vi "Knob Turn.vi"(0 "GEA2 Reference In":refnum<k24>, 7 "Knob Postiton":T1=enum."Position 1", 11 "Error In":errorcluster) -> (4 "GEA2 Reference Out":refnum<k24>, 15 "Error Out":errorcluster)   [LabVIEW 2016, in "TLMB.lvlib"]
uses:
  Projects/TLMB.lvlib
  type defs/Encoder Position.ctl
  Q:/Common/DLLs/GEA3/GeaCommunication.dll
  Common/DLLs/GEA3/GeaCommunication.dll
  Common/LabVIEW GEA2 Toolkit/LabVIEW_GEA2_Toolkit.lvlibp/type defs/Source_Destination.ctl
  Common/LabVIEW GEA2 Toolkit/LabVIEW_GEA2_Toolkit.lvlibp/type defs/ERD Write Data In.ctl
  Common/LabVIEW GEA2 Toolkit/LabVIEW_GEA2_Toolkit.lvlibp/type defs/Data Type.ctl
  Common/LabVIEW GEA2 Toolkit/LabVIEW_GEA2_Toolkit.lvlibp
panel:
  in  "Standalone?":bool
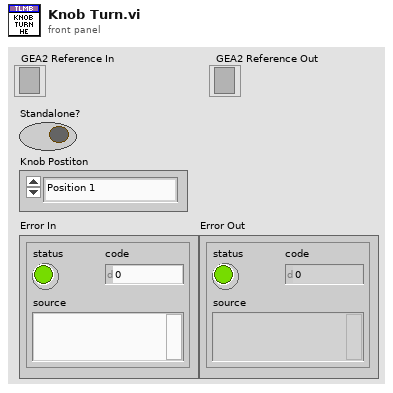
[diagram p1: front panel]
types:
  T1 = typedef "TLMB.lvlib/Encoder Position.ctl" = enum16{"Position 0", "Position 1", "Position 2", "Position 3", "Position 4", "Position 5", "Position 6", "Position 7", "Position 8", "Position 9", "Position 10", "Position 11", "Position 12", "Position 13", "Clear / Reset"}
  T2 = typedef "LabVIEW_GEA2_Toolkit.lvlibp/ERD Write Data In.ctl" = cluster{"ERD Number":u16, "Data Type":T3, "Data":string}
  T3 = typedef "LabVIEW_GEA2_Toolkit.lvlibp/Data Type.ctl" = enum16{"string", "boolean", "uint8_t", "uint16_t", "uint32_t", "uint64_t", "int8_t", "int16_t", "int32_t", "int64_t"}
  T4 = typedef "LabVIEW_GEA2_Toolkit.lvlibp/Source_Destination.ctl" = cluster{"Source":u8, "Destination":u8}
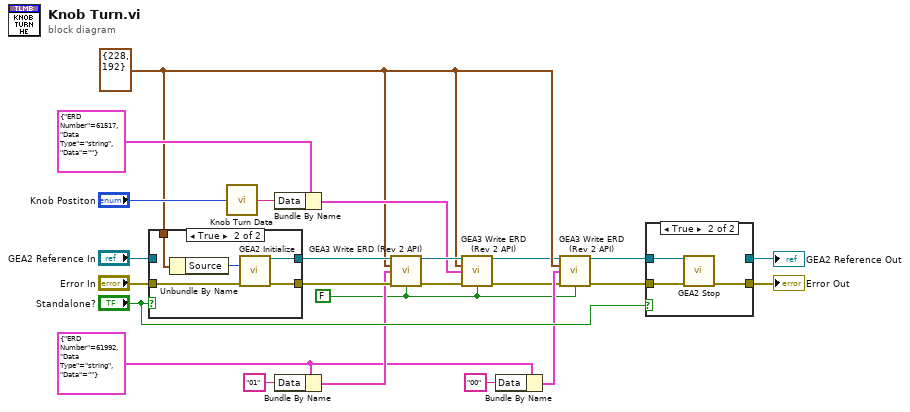
[diagram p0: block diagram]
diagram:
  w9 = T2 {"ERD Number"=61992, "Data Type"=enum."string", "Data"=""} ("ERD Write Data In")
  w4 = FALSE ("Verify ERD Response?")
  w3 = T4 {"Source"=228, "Destination"=192} ("GEA Inputs")
  n1 = case shown="True" "Standalone?" {
    tunnel: "Error In" -> [w25 w31]
    tunnel: [w25 w30] -> w17
    tunnel: "GEA2 Reference In" -> [w26 _]
    tunnel: [w26 w29] -> w18
    tunnel: w3 -> [_ w27]
    frame False {
    }
    frame True {
      n2 = Unbundle By Name(w27) -> ("Source"=w28:u8)
      n3 = call "GEA2 Initialize.vi"("Source Address"=w28, "error in"=w31) -> ("GEA2 Reference Out"=w29:refnum<k24>, "error out"=w30:errorcluster)  [unwired: 11 in, 1 out]
    }
  }
  n4 = call "Knob Turn Data.vi"("Switch"="Knob Postiton") -> ("Switch Message"=w6:string)  [unwired: 14 in]
  n5 = Bundle By Name(cluster=T2 {"ERD Number"=61517, "Data Type"=enum."string", "Data"=""} ("ERD Write Data In"), "Data"=w6) -> (w14:T2)
  n6 = Bundle By Name(cluster=w9, "Data"="01") -> (w12:T2)
  n7 = call "GEA3 Write ERD (Rev 2 API).vi"("GEA2 Reference In"=w18, "GEA Inputs"=w3, "ERD Write Data In"=w12, "Error In"=w17, "Verify ERD Response?"=w4) -> ("GEA2 Reference Out"=w16:refnum<k24>, "Error Out"=w15:errorcluster)  [unwired: 8 in, 1 out]
  n8 = call "GEA3 Write ERD (Rev 2 API).vi"("GEA2 Reference In"=w16, "GEA Inputs"=w3, "ERD Write Data In"=w14, "Error In"=w15, "Verify ERD Response?"=w4) -> ("GEA2 Reference Out"=w2:refnum<k24>, "Error Out"=w1:errorcluster)  [unwired: 8 in, 1 out]
  n9 = Bundle By Name(cluster=w9, "Data"="00") -> (w7:T2)
  n10 = call "GEA3 Write ERD (Rev 2 API).vi"("GEA2 Reference In"=w2, "GEA Inputs"=w3, "ERD Write Data In"=w7, "Error In"=w1, "Verify ERD Response?"=w4) -> ("GEA2 Reference Out"=w11:refnum<k24>, "Error Out"=w10:errorcluster)  [unwired: 8 in, 1 out]
  n11 = case shown="True" "Standalone?" {
    tunnel: [w32 w36] -> w21
    tunnel: w11 -> [w33 w35]
    tunnel: [w33 _] -> w20
    tunnel: w10 -> [w32 w34]
    frame False {
    }
    frame True {
      n12 = call "GEA2 Stop.vi"("GEA2 Reference In"=w35, "Error In"=w34) -> ("Error Out"=w36:errorcluster)  [unwired: 13 in]
    }
  }
  "Error Out" <- w21
  "GEA2 Reference Out" <- w20
